vi "適應性控制_輸入權重係數+數位積分_多頻率追蹤V3(實際控制).vi"() -> ()   [LabVIEW 2010]
panel:
  in  "pp":dbl
  in  "理想初始頻率":dbl=1.0
  in  "理想頻率數":i32=10
  in  "I增益":dbl
  out "當下誤差":dbl=0.1 format="%#_13g"
  out "模擬輸入x(t)":dbl[][](graph)
  in  "頻率間距":dbl=1.0
  out "理想與FIR輸出":dbl[][](graph)
  out "message":string=" INSTRUCTIONS:\r\rNormal Use:  When using subVIs that incorporate the error in/error out (or error I/O) structure, place this handler where you want to inform the user of an error, typically at the end of the I/O data path, as the last action of the program.  If the error in error? is ERROR, the handler creates a message describing the error and its source.  If the type of dialog = 1 (default), the message is displayed to the user, who can only acknowedge it.  If the type = 2, the user can acknowledge the message or abort execution; aborting a program with active I/O is not recommended.  If the type = 0, no message is displayed; this is used to process the error programmatically, and the error out cluster elements are wired to individual terminals for that reason.  \r\rOther Use:\n\r\nlocal testing.  To test the error code of a subVI or function that does not have the error I/O structure, you can wire its error code and a source string to the local error code and error source inputs.  If error in error? indicates no error and error code is not equal to 0, the local code and source are substituted for the error in values, and error? is set TRUE (ERROR)."
  out "誤差":dbl(graph)
  out "while平均運行時間":dbl
  out "收斂time":dbl
  out "各頻率誤差已達標準":bool
  in  "各頻率誤差低於多少亮燈":dbl=0.1 format="%#_13g"
  in  "理想振幅":dbl=0.2
  in  "理想直流偏移":dbl
  in  "理想相位(deg)":dbl
  in  "order":i32=100
  in  "取樣頻率":dbl=100.0 min=1.0 max=1000.0 step=1.0
  in  "stop":bool
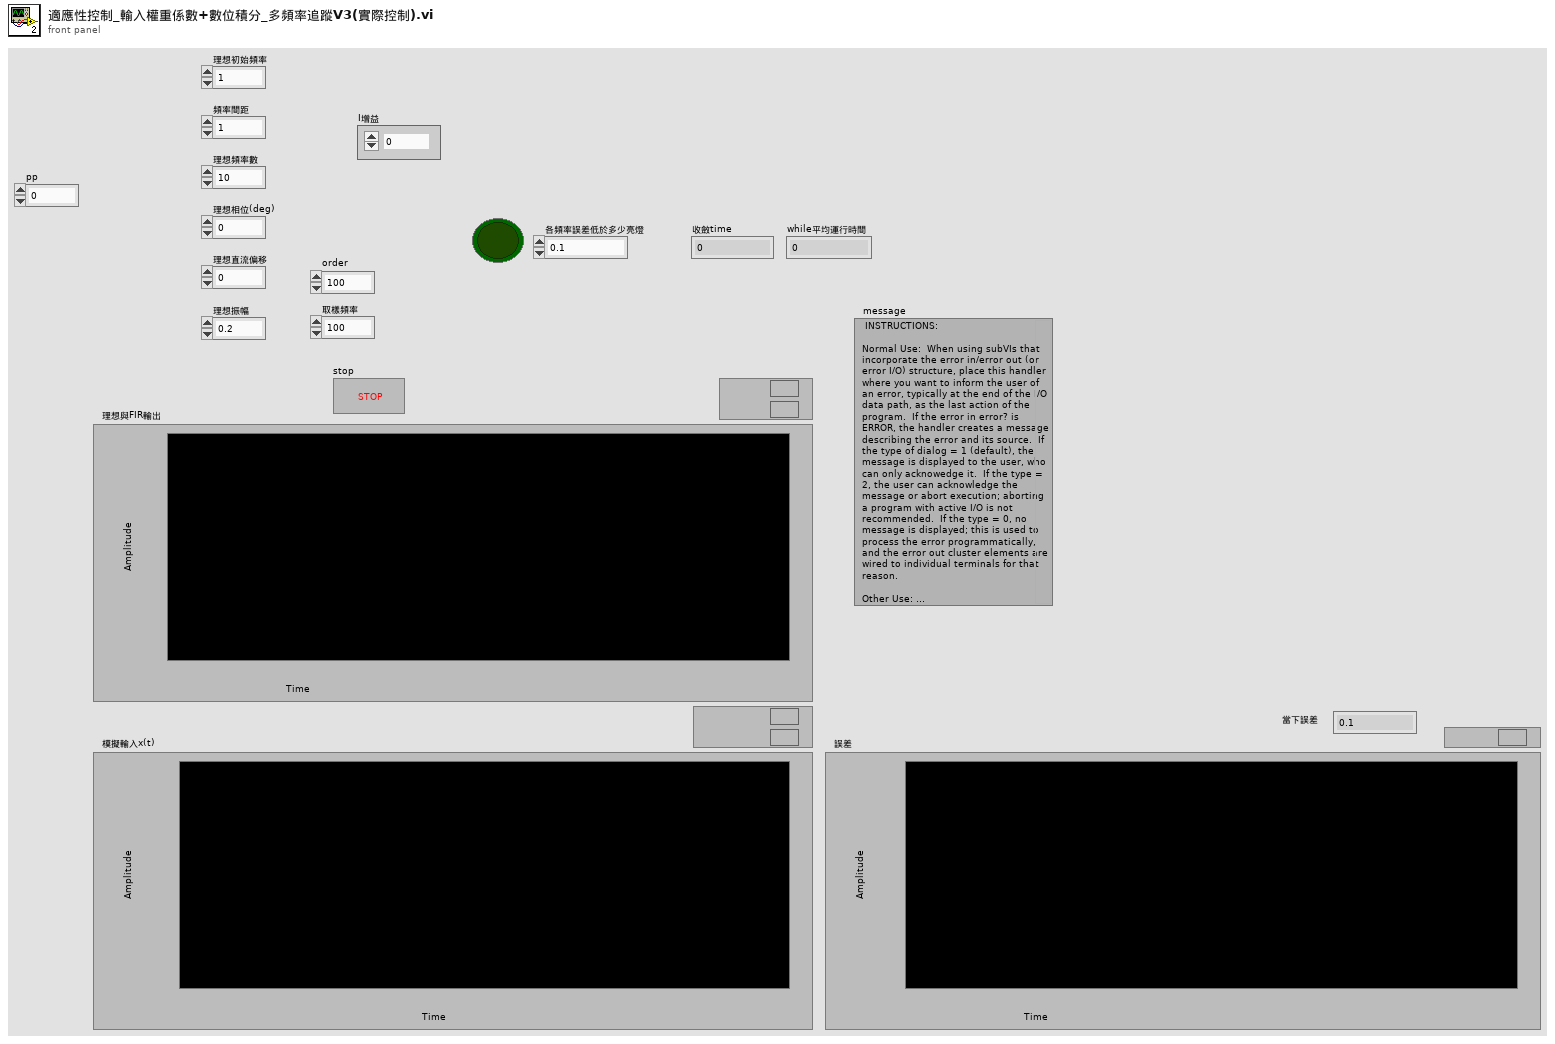
[diagram p1: front panel]
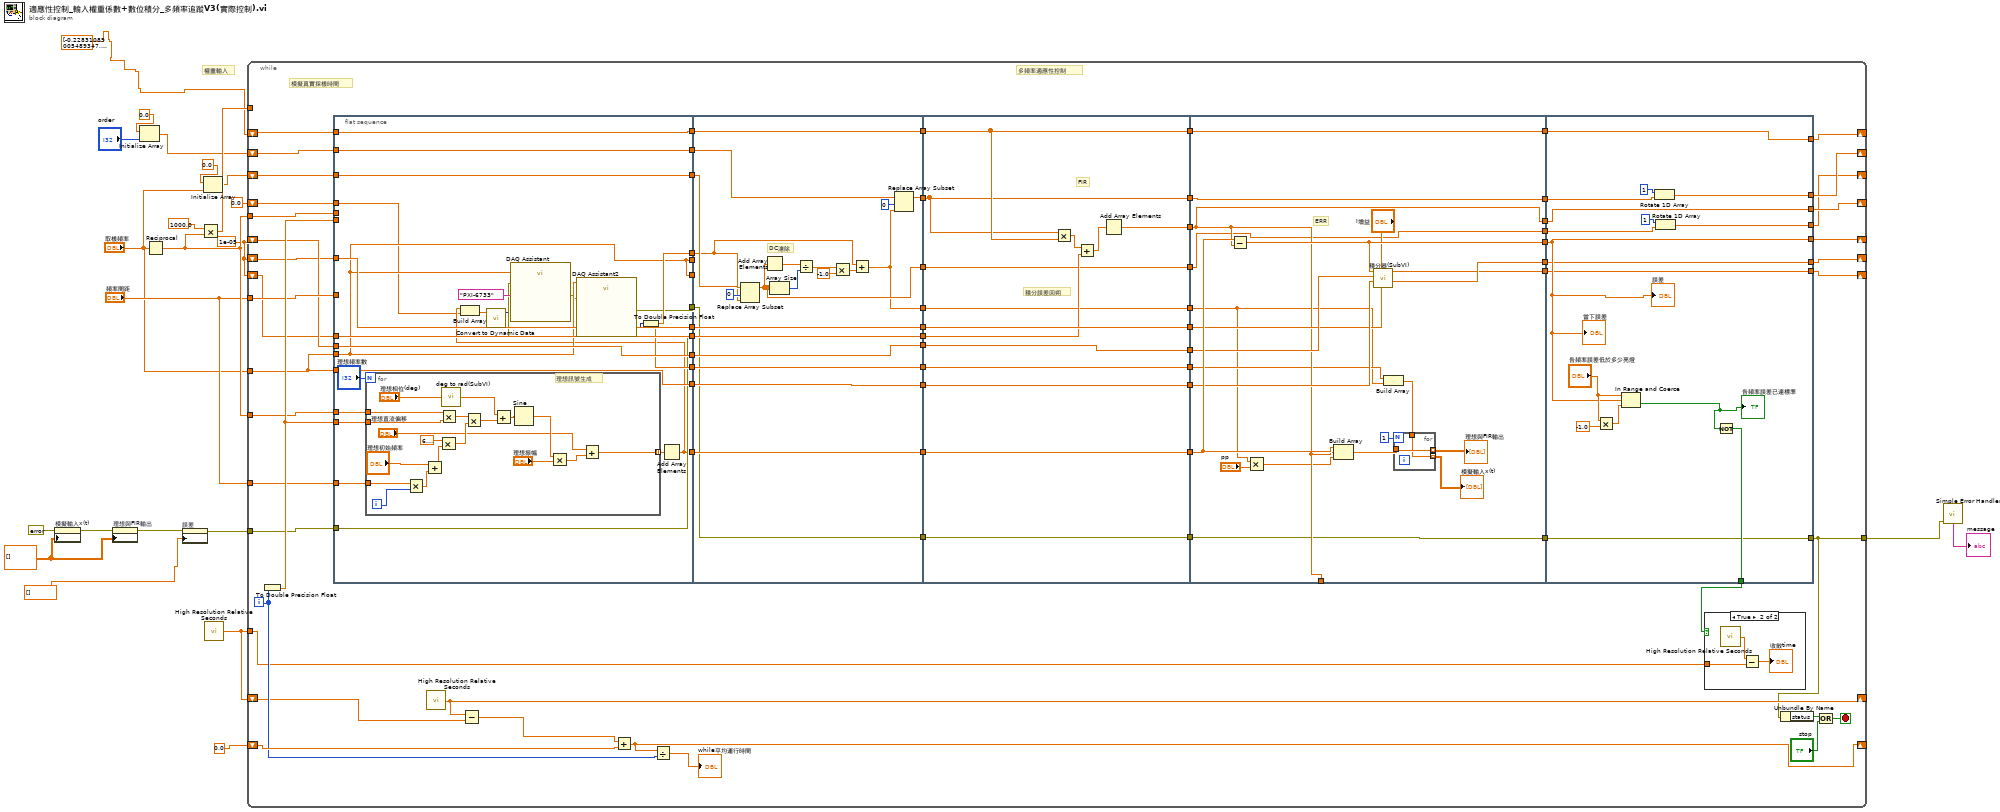
[diagram p0: block diagram]
diagram:
  w10 = 1e-05 ("x")
  w3 = dbl[][] [] ("History Data")
  # "權重輸入"
  n1 = property on="模擬輸入x(t)" class="WFChart (strict)"(error in=errorcluster {"status"=FALSE, "code"=0, "source"=""} ("error constant"), "History Data"=w3) -> (error out=w14:errorcluster)  [unwired: 1 in, 1 out]
  n2 = property on="理想與FIR輸出" class="WFChart (strict)"(error in=w14, "History Data"=w3) -> (error out=w15:errorcluster)  [unwired: 1 in, 1 out]
  n3 = Initialize Array(0.0 ("element"), "order") -> (w8:dbl[])
  n4 = Reciprocal(x="取樣頻率") -> (1/x=w22:dbl)
  n5 = property on="誤差" class="WFChart (strict)"(error in=w15, "History Data"=dbl[] []) -> (error out=w17:errorcluster)  [unwired: 1 in, 1 out]
  n6 = Multiply(x=1000.0, y=w22) -> (x*y=w20:dbl)
  n7 = Initialize Array(0.0 ("element"), "取樣頻率") -> (w5:dbl[])
  n8 = call <vilib>:"High Resolution Relative Seconds.vi"() -> ("relative seconds"=w19:dbl)
  n9 = while {
    shift-right: [w67] -> _
    shift-left: w8 -> [w99]
    shift-right: [w65] -> _
    shift-left: dbl[] [-0.22831089005489347, -0.2535548147535409, -0.27487188372126353, -0.291976070033387, -0.30462466208407313, -0.31266654951885986, -0.31599111399379676, -0.3145636637066062, -0.3084245103884838, -0.2976771791349662, -0.28249110611392697, -0.26310447975386503, -0.23981649771765953, -0.21297651003446433, -0.1829884241357615, -0.150303471707352, -0.11540716466795142, -0.07881610610589203, -0.04107659847119702, -0.002754947823625345] ("權重(w)") -> [w94]
    tunnel: w22 -> [w85]
    tunnel: w22 -> [w84]
    tunnel: w20 -> [_]
    tunnel: w19 -> [w76]
    shift-right: [w77] -> _
    shift-left: w19 -> [w75]
    shift-right: [w78] -> _
    shift-left: 0.0 -> [w80]
    tunnel: w17 -> [w72]
    tunnel: "頻率間距" -> [w71]
    shift-right: [w64] -> _
    shift-left: w10 -> [w60]
    shift-right: [w56] -> _
    shift-left: w10 -> [w51]
    shift-right: [w50] -> _
    shift-left: w10 -> [w46]
    tunnel: "取樣頻率" -> [w44]
    tunnel: "頻率間距" -> [w45]
    shift-right: [w39] -> _
    shift-left: 0.0 -> [w38]
    shift-right: [w32] -> _
    shift-left: w5 -> [w37]
    tunnel: [w24] -> w2
    i -> [w79]
    stop <- w27 stop-if-true
    # "模擬真實採樣時間"
    # "多頻率適應性控制"
    n10 = To Double Precision Float(number=w79) -> (double precision float=w92:dbl)
    n11 = flat-sequence {
      tunnel: w92 -> [_]
      tunnel: [w126] -> w100
      tunnel: w99 -> [w126]
      tunnel: [w114] -> w98
      tunnel: [w125] -> w95
      tunnel: w94 -> [w125]
      tunnel: w92 -> [w124]
      tunnel: [w108] -> w89
      tunnel: w85 -> [_]
      tunnel: w84 -> [w123]
      tunnel: w72 -> [w111]
      tunnel: w71 -> [_]
      tunnel: [w114] -> w68
      tunnel: [w122] -> w61
      tunnel: w60 -> [w122]
      tunnel: [w121] -> w57
      tunnel: w44 -> [w121]
      tunnel: [w120] -> w52
      tunnel: w51 -> [w120]
      tunnel: [w119] -> w47
      tunnel: w46 -> [w119]
      tunnel: w45 -> [w117]
      tunnel: w44 -> [w113]
      tunnel: [w113] -> w43
      tunnel: [w113] -> w42
      tunnel: [w109] -> w41
      tunnel: w38 -> [w107]
      tunnel: w37 -> [w104]
      tunnel: [w104] -> w36
      tunnel: w100 -> [w164]
      tunnel: w98 -> [w147]
      tunnel: [w156] -> w97
      tunnel: [w166] -> w96
      tunnel: w95 -> [w166]
      tunnel: [w165] -> w90
      tunnel: w89 -> [w165]
      tunnel: [w157] -> w73
      tunnel: [w163] -> w69
      tunnel: w68 -> [w163]
      tunnel: [w161] -> w62
      tunnel: w61 -> [w161]
      tunnel: [w160] -> w58
      tunnel: w57 -> [w160]
      tunnel: [w159] -> w53
      tunnel: w52 -> [w159]
      tunnel: [w158] -> w48
      tunnel: w47 -> [w158]
      tunnel: w43 -> [_]
      tunnel: w42 -> [_]
      tunnel: w41 -> [w157]
      tunnel: w36 -> [w154]
      tunnel: [w148] -> w35
      tunnel: [w146] -> w25
      tunnel: w97 -> [w178]
      tunnel: w96 -> [w180]
      tunnel: [w180] -> w93
      tunnel: [w171] -> w91
      tunnel: w90 -> [w171]
      tunnel: [w170] -> w88
      tunnel: [w178] -> w87
      tunnel: w73 -> [w168]
      tunnel: [w179] -> w70
      tunnel: w69 -> [w179]
      tunnel: [w177] -> w63
      tunnel: w62 -> [w177]
      tunnel: [w176] -> w59
      tunnel: w58 -> [w176]
      tunnel: [w175] -> w54
      tunnel: w53 -> [w175]
      tunnel: w48 -> [w173]
      tunnel: w35 -> [w169]
      tunnel: [w169] -> w34
      tunnel: [w168] -> w30
      tunnel: [w167] -> w26
      tunnel: w25 -> [w167]
      tunnel: w93 -> [w196]
      tunnel: w91 -> [w197]
      tunnel: w88 -> [w188]
      tunnel: w87 -> [w199]
      tunnel: [w199] -> w86
      tunnel: [w194] -> w83
      tunnel: w70 -> [w185]
      tunnel: [w196] -> w66
      tunnel: w63 -> [w195]
      tunnel: w59 -> [w193]
      tunnel: [w191] -> w55
      tunnel: w54 -> [w190]
      tunnel: [w189] -> w49
      tunnel: [w188] -> _
      tunnel: [w188] -> w40
      tunnel: w34 -> [w187]
      tunnel: [w187] -> w33
      tunnel: [w186] -> w31
      tunnel: w30 -> [w186]
      tunnel: w26 -> [w182]
      tunnel: w86 -> [w215]
      tunnel: [w221] -> w67
      tunnel: w83 -> [w212]
      tunnel: [w217] -> w74
      tunnel: [w213] -> w65
      tunnel: w66 -> [w213]
      tunnel: [w212] -> w64
      tunnel: [w211] -> w56
      tunnel: w55 -> [w211]
      tunnel: [w210] -> w50
      tunnel: w49 -> [w210]
      tunnel: w40 -> [w209]
      tunnel: [w209] -> w39
      tunnel: w33 -> [w207]
      tunnel: [w206] -> w32
      tunnel: [w205] -> w24
      tunnel: w31 -> [w205]
      frame #0 {
        n12 = for {
          N: "理想頻率數" -> [_]
          tunnel: w124 -> [w145]
          tunnel: [w144] -> w116 mode=indexing
          tunnel: w123 -> [w143]
          tunnel: w117 -> [w129]
          i -> [w130]
          # "理想訊號生成"
          n13 = Multiply(x=w129, y=w130) -> (x*y=w131:dbl)
          n14 = Add(x="理想初始頻率", y=w131) -> (x+y=w127:dbl)
          n15 = Multiply(x=6.283185307179586, y=w127) -> (x*y=w140:dbl)
          n16 = Multiply(x=w143, y=w145) -> (x*y=w133:dbl)
          n17 = call "deg to rad(SubVI).vi"("Degree"="理想相位(deg)") -> ("Radian"=w137:dbl)
          n18 = Multiply(x=w133, y=w140) -> (x*y=w141:dbl)
          n19 = Add(x=w137, y=w141) -> (x+y=w142:dbl)
          n20 = Sine(x=w142) -> (sin(x)=w138:dbl)
          n21 = Multiply(x=w138, y="理想振幅") -> (x*y=w139:dbl)
          n22 = Add(x="理想直流偏移", y=w139) -> (x+y=w144:dbl)
        }
        n23 = Add Array Elements(numeric array=w116) -> (sum=w108:dbl)
        n24 = Build Array(w108, w107) -> (w106:dbl[])
        n25 = call "Convert to Dynamic Data"("Array"=w106) -> ("Dynamic Data Type"=w105:dynamicdata)  [unwired: 3 in]
        n26 = call "DAQ Assistant"("data"=w105, "rate"=w113, "error in"=w111, "device name"=tag "PXI-6733") -> ("error out"=w110:errorcluster)  [unwired: 13 in, 2 out]
        n27 = call "DAQ Assistant2"("rate"=w113, "error in"=w110) -> ("data"=w115:dynamicdata, "error out"=w109:errorcluster)  [unwired: 14 in, 2 out]
        n28 = To Double Precision Float(number=w115) -> (double precision float=w114:dbl)
      }
      frame #1 {
        # "DC濾除"
        n29 = Replace Array Subset(array=w154, new element=w147, index=0) -> (w148:dbl[])
        n30 = Add Array Elements(numeric array=w148) -> (sum=w153:dbl)
        n31 = Array Size(array=w148) -> (size(s)=w152:i32)
        n32 = Divide(x=w153, y=w152) -> (x/y=w151:dbl)
        n33 = Multiply(x=w151, y=-1.0) -> (x*y=w149:dbl)
        n34 = Add(x=w147, y=w149) -> (x+y=w146:dbl)
        n35 = Replace Array Subset(array=w164, new element=w146, index=0) -> (w156:dbl[])
      }
      frame #2 {
        # "積分誤差回朔"
        # "FIR"
        n36 = Multiply(x=w178, y=w180) -> (x*y=w174:dbl[])
        n37 = Add(x=w174, y=w173) -> (x+y=w172:dbl[])
        n38 = Add Array Elements(numeric array=w172) -> (sum=w170:dbl)
      }
      frame #3 {
        # "ERR"
        n39 = Subtract(x=w197, y=w188) -> (x-y=w194:dbl)
        n40 = Multiply(x=w182, y="pp") -> (x*y=w181:dbl)
        n41 = Build Array(w197, w188, w181) -> (w201:dbl[])
        n42 = call "積分器(SubVI).vi"("輸入累加ERR回朔"=w190, "I增益"="I增益", "samples (Hz)"=w193, "前一個ERR"=w195, "當下ERR"=w194) -> ("輸出累加ERR回朔"=w191:dbl, "積分修正量"=w189:dbl)  [unwired: 5 in]
        n43 = Build Array(w185, w182) -> (w184:dbl[])
        n44 = for {
          N: 1 -> [_]
          tunnel: [w204] -> w198 mode=indexing
          tunnel: w201 -> [w204]
          tunnel: [w203] -> w200 mode=indexing
          tunnel: w184 -> [w203]
        }
        "理想與FIR輸出" <- w198
        "模擬輸入x(t)" <- w200
      }
      frame #4 {
        n45 = Multiply(x="各頻率誤差低於多少亮燈", y=-1.0) -> (x*y=w218:dbl)
        n46 = In Range and Coerce(upper limit="各頻率誤差低於多少亮燈", x=w212, lower limit=w218) -> (In Range?=w214:bool)  [unwired: 1 out]
        "各頻率誤差已達標準" <- w214
        n47 = Rotate 1D Array(1:w215, 2:1 ("n")) -> (0:w221:dbl[])
        n48 = Rotate 1D Array(1:w207, 2:1 ("n")) -> (0:w206:dbl[])
        n49 = Not(x=w214) -> (.not. x?=w217:bool)
        "誤差" <- w212
        "當下誤差" <- w212
      }
    }
    n50 = call <vilib>:"High Resolution Relative Seconds.vi"() -> ("relative seconds"=w77:dbl)
    n51 = Subtract(x=w77, y=w75) -> (x-y=w82:dbl)
    n52 = Add(x=w82, y=w80) -> (x+y=w78:dbl)
    n53 = Divide(x=w78, y=w79) -> (x/y=→"while平均運行時間":dbl)
    n54 = case shown="True" w74 {
      tunnel: w76 -> [_ w101]
      frame False {
      }
      frame True {
        n55 = call <vilib>:"High Resolution Relative Seconds.vi"() -> ("relative seconds"=w103:dbl)
        n56 = Subtract(x=w103, y=w101) -> (x-y=→"收斂time":dbl)
      }
    }
    n57 = Unbundle By Name(w24) -> ("status"=w29:bool)
    n58 = Or(x=w29, y="stop") -> (x .or. y?=w27:bool)
  }
  n59 = call <vilib>:"Simple Error Handler.vi"("error in (no error)"=w2) -> ("message"=→"message":string)  [unwired: 4 in, 4 out]
